vi "areOverlapped.vi"(8 "error in (no error)":errorcluster, 10 "GObject2":refnum<class "GObject.lvclass">, 11 "GObject1":refnum<class "GObject.lvclass">) -> (0 "error out":errorcluster, 1 "areObjectsOverlapped?":bool, 2 "GObject2(dup)":refnum<class "GObject.lvclass">, 3 "GObject1(dup)":refnum<class "GObject.lvclass">)   [LabVIEW 2023, in "TLC_Scripto.lvlib"]
uses:
  TLC_Scripto.lvlib
  GObject/GObject.lvclass
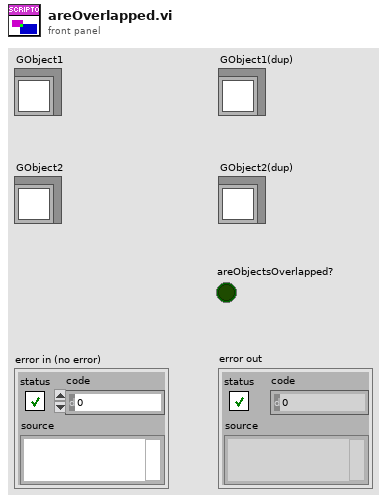
[diagram p1: front panel]
types:
  T1 = typedef "TLC_Scripto.lvlib/rectangle.ctl" = cluster{"left":i32, "top":i32, "right":i32, "bottom":i32}
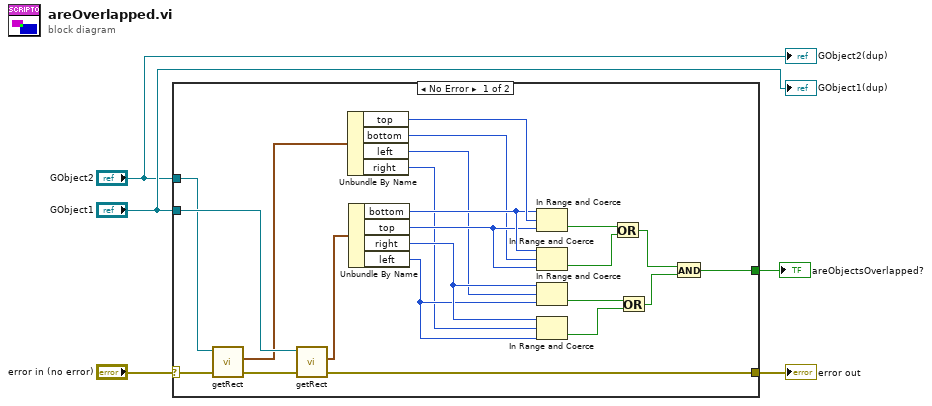
[diagram p0: block diagram]
diagram:
  n1 = case shown="No Error" "error in (no error)" {
    selector: "error in (no error)" -> [w22 w28]
    tunnel: "GObject1" -> [w27 _]
    tunnel: [w26 w28] -> w4
    tunnel: "GObject2" -> [w25 _]
    tunnel: [w6 _] -> w1
    frame No Error {
      n2 = call-dynamic "getRect.vi"("error in (no error)"=w22, "GObject in"=w25) -> ("error out"=w21:errorcluster, "rectangle"=w23:T1)  [unwired: 7 in, 1 out]
      n3 = call-dynamic "getRect.vi"("error in (no error)"=w21, "GObject in"=w27) -> ("error out"=w26:errorcluster, "rectangle"=w24:T1)  [unwired: 7 in, 1 out]
      n4 = Unbundle By Name(w23) -> ("top"=w20:i32, "bottom"=w17:i32, "left"=w14:i32, "right"=w13:i32)
      n5 = Unbundle By Name(w24) -> ("bottom"=w19:i32, "top"=w18:i32, "right"=w16:i32, "left"=w15:i32)
      n6 = In Range and Coerce(upper limit=w19, x=w20, lower limit=w18) -> (In Range?=w12:bool)  [unwired: 1 out]
      n7 = In Range and Coerce(upper limit=w19, x=w17, lower limit=w18) -> (In Range?=w11:bool)  [unwired: 1 out]
      n8 = In Range and Coerce(upper limit=w16, x=w14, lower limit=w15) -> (In Range?=w10:bool)  [unwired: 1 out]
      n9 = In Range and Coerce(upper limit=w16, x=w13, lower limit=w15) -> (In Range?=w9:bool)  [unwired: 1 out]
      n10 = Or(x=w12, y=w11) -> (x .or. y?=w8:bool)
      n11 = Or(x=w10, y=w9) -> (x .or. y?=w7:bool)
      n12 = And(x=w8, y=w7) -> (x .and. y?=w6:bool)
    }
    frame Error {
    }
  }
  "error out" <- w4
  "areObjectsOverlapped?" <- w1
  "GObject1(dup)" <- "GObject1"
  "GObject2(dup)" <- "GObject2"
